vi "AnalyzeVIs--function.vi"(6 "Report Save Type (ASCII)":u16(ring)=1 items=["ASCII", "HTML", "RSL File"], 7 "ReportPath":path=path "C:/Users/pauloneill/SCC/Orion/LabVIEW/VIAnalyzerOutput/manual", 8 "error in":errorcluster, 9 "Configuration File Password":string, 10 "VIANConfig":path=path "C:/Users/pauloneill/SCC/Orion/LabVIEW/Tests/Static/minimal.viancfg", 11 "VIs to Analyze":path[](array[path])=[path "C:/Users/pauloneill/SCC/Orion/LabVIEW/Source/App/Startup.vi"]) -> (0 "error out":errorcluster, 3 "Summary Statistics":T1={"Passed Tests"=39, "Failed Tests"=4, "Skipped Tests"=0, "VIs not loadable"=0, "Tests not loadable"=0, "Tests not runnable"=0, "Test error out"=0, "Start Time"=3753998548, "Total Time (s)"=91.253})   [LabVIEW 2020, in "CICD.lvlib"]
doc: "Run VI Analyzer on an array of input VIs and report summary statistics."
uses:
  CICD.lvlib
  <vilib>/addons/analyzer/_vianresshared.llb/VIAnRes Export Options.ctl
  <vilib>/addons/analyzer/NI_VIAnalyzerTKVIs.lvlib
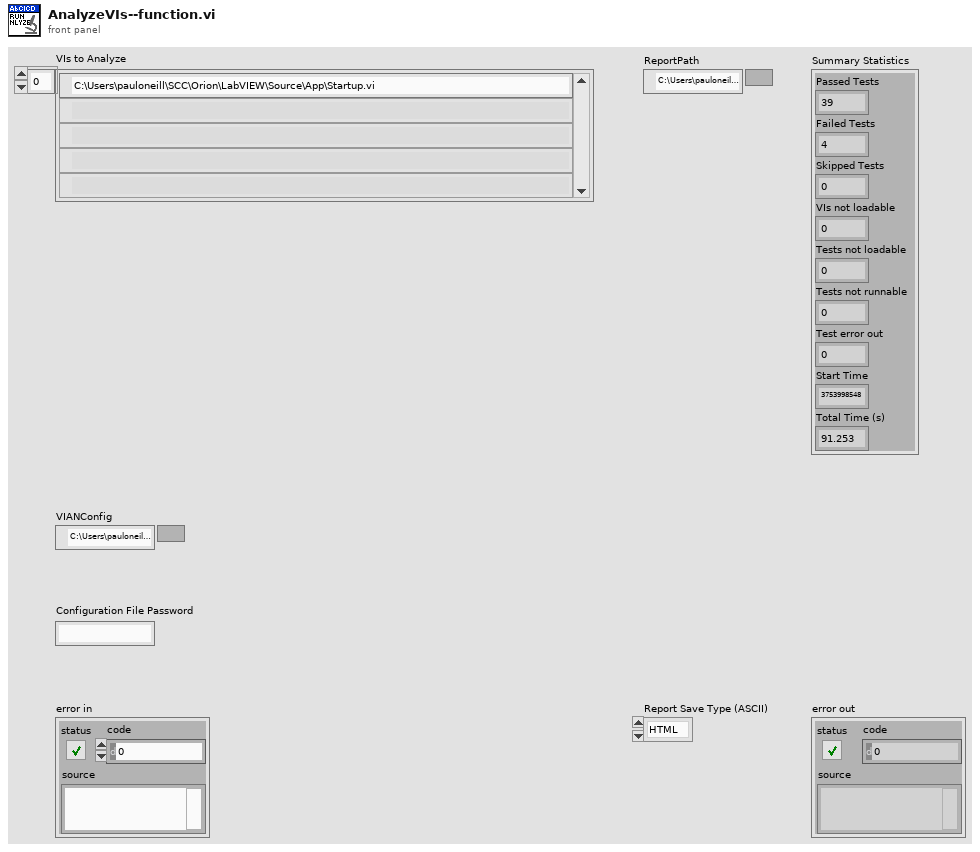
[diagram p1: front panel]
types:
  T1 = cluster{"Passed Tests":i32, "Failed Tests":i32, "Skipped Tests":i32, "VIs not loadable":i32, "Tests not loadable":i32, "Tests not runnable":i32, "Test error out":i32, "Start Time":u32, "Total Time (s)":dbl}
  T2 = typedef "VIAnRes Export Options.ctl" = cluster{"Summary Data":bool, "Failed Tests":bool, "Passed Tests":bool, "Skipped Tests":bool, "Errors":bool}
  T3 = typedef "VIAnAPI Ref.ctl" = refnum<k1>
  T4 = typedef "VIAnCtl Results.ctl" = cluster{"Test Name":string, "Results Data":T5[], "Status":T6, "Exceed Max Fails?":bool}
  T5 = typedef "VIAnCtl ResultsData (index).ctl" = cluster{"Result Message":string, "Ref Index":i32}
  T6 = typedef "VIAnCtl ResultStatus.ctl" = enum16{"Pass", "Fail", "Skipped", "VI not loadable", "Test not loadable", "Test not runnable", "Test error out"}
  T7 = typedef "VIAnRes Parsed Results Data (by VI).ctl" = cluster{"VI Path":path, "Pass":cluster{"row":i32, "column":i32}[], "Fail":cluster{"row":i32, "column":i32}[], "Skipped":cluster{"row":i32, "column":i32}[], "VI not loadable":cluster{"row":i32, "column":i32}[], "Test not loadable":cluster{"row":i32, "column":i32}[], "Test not runnable":cluster{"row":i32, "column":i32}[], "Test error out":cluster{"row":i32, "column":i32}[]}
  T8 = typedef "VIAnRes Parsed Results Data (by Test).ctl" = cluster{"Test Name":string, "Pass":cluster{"VI Path":path, "index":cluster{"row":i32, "column":i32}}[], "Fail":cluster{"VI Path":path, "index":cluster{"row":i32, "column":i32}}[], "Skipped":cluster{"VI Path":path, "index":cluster{"row":i32, "column":i32}}[]}
  T9 = typedef "VIAnCtl Test Config Data.ctl" = cluster{"Test Name":string, "Config Ref":refnum<vi>, "Ref Valid?":bool, "Test Ranking":T10, "Max Failures":u32, "Test Path":path, "Control Values":T11[], "Selected?":bool}
  T10 = typedef "VIAnCtl TestRanking.ctl" = u16
  T11 = typedef "VIAnCtl Config Control Value.ctl" = cluster{"Control Name":string, "Control Value":variant}
  T12 = cluster{"Raw Results":T4[][], "Parsed Results Data (by VI)":T7[], "Parsed Results Data (by Test)":T8[], "Summary Statistics":cluster{"Passed Tests":i32, "Failed Tests":i32, "Skipped Tests":i32, "VIs not loadable":i32, "Tests not loadable":i32, "Tests not runnable":i32, "Test error out":i32, "Start Time":u32, "Total Time (s)":dbl}, "Test Config Data":T9[]}
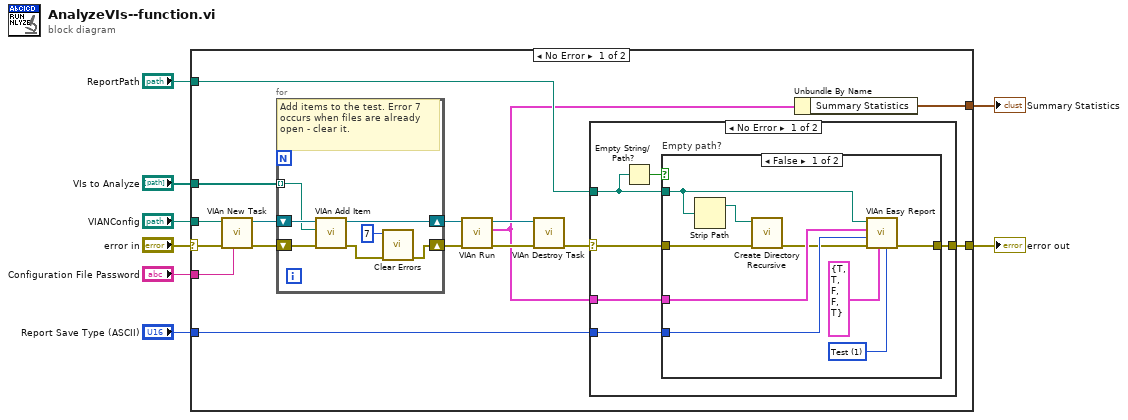
[diagram p0: block diagram]
diagram:
  n1 = case shown="No Error" "error in" {
    selector: "error in" -> [w19 w49]
    tunnel: [w20 w49] -> w8
    tunnel: "VIANConfig" -> [w18 _]
    tunnel: "VIs to Analyze" -> [w14 _]
    tunnel: "ReportPath" -> [w13 _]
    tunnel: "Configuration File Password" -> [w12 _]
    tunnel: [w10 _] -> w2
    tunnel: "Report Save Type (ASCII)" -> [w9 _]
    frame No Error {
      n2 = call <vilib>:"VIAn New Task.vi"("Configuration File Password"=w12, "error in (no error)"=w19, "Path to Configuration File"=w18) -> ("error out"=w22:errorcluster, "VI Analyzer Task"=w16:T3)  [unwired: 7 in]
      n3 = for {
        shift-right: [w46] -> w24
        shift-left: w22 -> [w48]
        shift-right: [w44] -> w17
        shift-left: w16 -> [w45]
        tunnel: w14 -> [w43] mode=indexing
        # "Add items to the test. Error 7 occurs when files are already open - clear it."
        n4 = call <vilib>:"VIAn Add Item.vi"("error in (no error)"=w48, "Item to Add"=w43, "VI Analyzer Task in"=w45) -> ("error out"=w47:errorcluster, "VI Analyzer Task out"=w44:T3)  [unwired: 7 in]
        n5 = call <vilib>:"Clear Errors.vi"("error in (no error)"=w47, "specific error code to clear (0: all)"=7) -> ("error out"=w46:errorcluster)  [unwired: 4 in, 1 out]
      }
      n6 = call <vilib>:"VIAn Run.vi"("error in (no error)"=w24, "VI Analyzer Task in"=w17) -> ("error out"=w23:errorcluster, "Analysis Results"=w11:T12, "VI Analyzer Task out"=w15:T3)  [unwired: 5 in, 2 out]
      n7 = call <vilib>:"VIAn Destroy Task.vi"("error in (no error)"=w23, "VI Analyzer Task in"=w15) -> ("error out"=w21:errorcluster)  [unwired: 9 in]
      n8 = case shown="No Error" w21 {
        selector: w21 -> [w30 w41]
        tunnel: w11 -> [w28 _]
        tunnel: [w29 w41] -> w20
        tunnel: w13 -> [w25 _]
        tunnel: w9 -> [w27 _]
        frame No Error {
          n9 = Empty String/Path?(string/path=w25) -> (empty?=w26:bool)
          n10 = case "Empty path?" shown="False" w26 {
            tunnel: w30 -> [w31 w40]
            tunnel: [w39 w40] -> w29
            tunnel: w28 -> [w38 _]
            tunnel: w25 -> [w34 _]
            tunnel: w27 -> [w35 _]
            frame False {
              w36 = u16 1 items=["VI", "Test"] ("Sort Type (VI)")
              n11 = Strip Path(path=w34) -> (stripped path=w33:path)  [unwired: 1 out]
              n12 = call <vilib>:"Create Directory Recursive.vi"("error in (no error)"=w31, "directory"=w33) -> ("error out"=w32:errorcluster)  [unwired: 3 in, 2 out]
              n13 = call <vilib>:"VIAn Easy Report.vi"("Sort Type (VI)"=w36, "Export Options (Summary, Fails, Errs)"=T2 {"Summary Data"=TRUE, "Failed Tests"=TRUE, "Passed Tests"=FALSE, "Skipped Tests"=FALSE, "Errors"=TRUE}, "error in (no error)"=w32, "Report Save Type (ASCII)"=w35, "Analysis Results"=w38, "Report Save Path"=w34) -> ("error out"=w39:errorcluster)  [unwired: 5 in]
            }
            frame True {
            }
          }
        }
        frame Error {
        }
      }
      n14 = Unbundle By Name(w11) -> ("Summary Statistics"=w10:T1)
    }
    frame Error {
    }
  }
  "error out" <- w8
  "Summary Statistics" <- w2
